vi "Configure Std Waveform.vi"(8 "error in (no error)":errorcluster, 11 "FGen PXI Base CFG in":refnum<class "FGen PXI Base CFG.lvclass">) -> (0 "error out":errorcluster, 3 "FGen PXI Base CFG out":refnum<class "FGen PXI Base CFG.lvclass">)   [LabVIEW 2023, in "FGen PXI Base CFG.lvlib" / "FGen PXI Base CFG.lvclass"]
uses:
  FGen PXI Base CFG.lvclass
  <instrlib>/niFgen/niFgen.llb/niFgen Waveform Type.ctl
  <instrlib>/niFgen/niFgen.llb/niFgen Trigger Mode.ctl
  <instrlib>/niFgen/niFgen.llb/niFgen Output Impedance.ctl
  FGen PXI Base CFG.lvclass/FGen PXI Base CFG.ctl
  Configuration/Configuration JSON/Configuration JSON Base/CFG JSON.lvclass/CFG JSON.ctl
  <instrlib>/niFgen/niFgen.llb/niFgen Output Mode.ctl
  ad788453-c75c-4861-a618-ce10b1873926.vi
  <vilib>/JDP Science/JSONtext/Find Item.vi
  <vilib>/JDP Science/JSONtext/Next JSON Value.vi
  <vilib>/JDP Science/JSONtext/String Subset.vi
  <vilib>/JDP Science/JSONtext/Parsing/Advance past next JSON Value (inlined COPY).vi
  <vilib>/JDP Science/JSONtext/Parsing/Advance past whitespace.vi
  <vilib>/JDP Science/JSONtext/Parsing/Advance past String.vi
  <vilib>/JDP Science/JSONtext/Parsing/Advance past Number.vi
  <vilib>/JDP Science/JSONtext/Parsing/Advance past Line Ending.vi
  <vilib>/JDP Science/JSONtext/Parsing/Parse Full Path or Item Name.vi
  <vilib>/JDP Science/JSONtext/Parsing/Advance past Array.vi
  <vilib>/JDP Science/JSONtext/Parsing/Advance past Object.vi
  <vilib>/JDP Science/JSONtext/support/Error Cluster From Code.vi
  <vilib>/JDP Science/JSONtext/Offset/Find Item Locations by Path.vi
  <vilib>/JDP Science/JSONtext/JSON text to Variant.vi
  <vilib>/Utility/error.llb/Error Cluster From Error Code.vi
  <vilib>/JDP Science/JSONtext/LVClass Serializer/JSONtext LVClass Serializer.lvclass
  <vilib>/ErrorRing/Error Ring.xnode
  Configuration/Configuration JSON/Configuration JSON Base/CFG JSON.lvclass
  D:/git/HAL/HAL GOOP4/FGen/FGen Base CFG/FGen Base CFG.lvclass
  D:/git/HAL/HAL GOOP4/Configuration/Configuration JSON/Configuration JSON Base/CFG JSON.lvclass
  D:/git/HAL/HAL GOOP4/Interfaces/IConfigure/IConfigure.lvclass
  D:/git/HAL/HAL GOOP4/FGen/FGen PXI/FGen PXI Base CFG/FGen PXI Base CFG.lvclass
panel:
  out "Impedance":T1 caption="Impedance (default: 0=50 ohms)" items=["50 ohms", "75 ohms"]
  out "Trigger Mode":T2 caption="Trigger Mode (default: 1=continuous)" items=["Single", "Continuous", "Stepped", "Burst"]
  out "Waveform":T3 items=["Sine", "Square", "Triangle", "Ramp Up", "Ramp Down", "DC", "Noise", "User"]
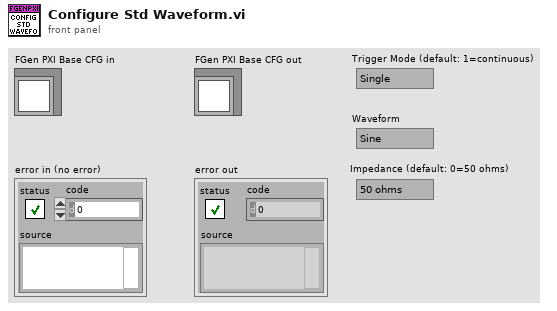
[diagram p1: front panel]
types:
  T1 = typedef "niFgen Output Impedance.ctl" = i32
  T2 = typedef "niFgen Trigger Mode.ctl" = i32
  T3 = typedef "niFgen Waveform Type.ctl" = i32
  T4 = cluster{"Name":string, "Enabled":bool, "Waveform":string, "Frequency":dbl, "Amplitude":dbl, "Start Phase":dbl, "DC Offset":dbl, "Trigger Mode":string, "Impedance":string}[]
  T5 = typedef "niFgen Output Mode.ctl" = u32
  T6 = typedef "LVStringsAndValuesArrayTypeDef_I32.ctl" = cluster{"String":string, "Value":i32}[]
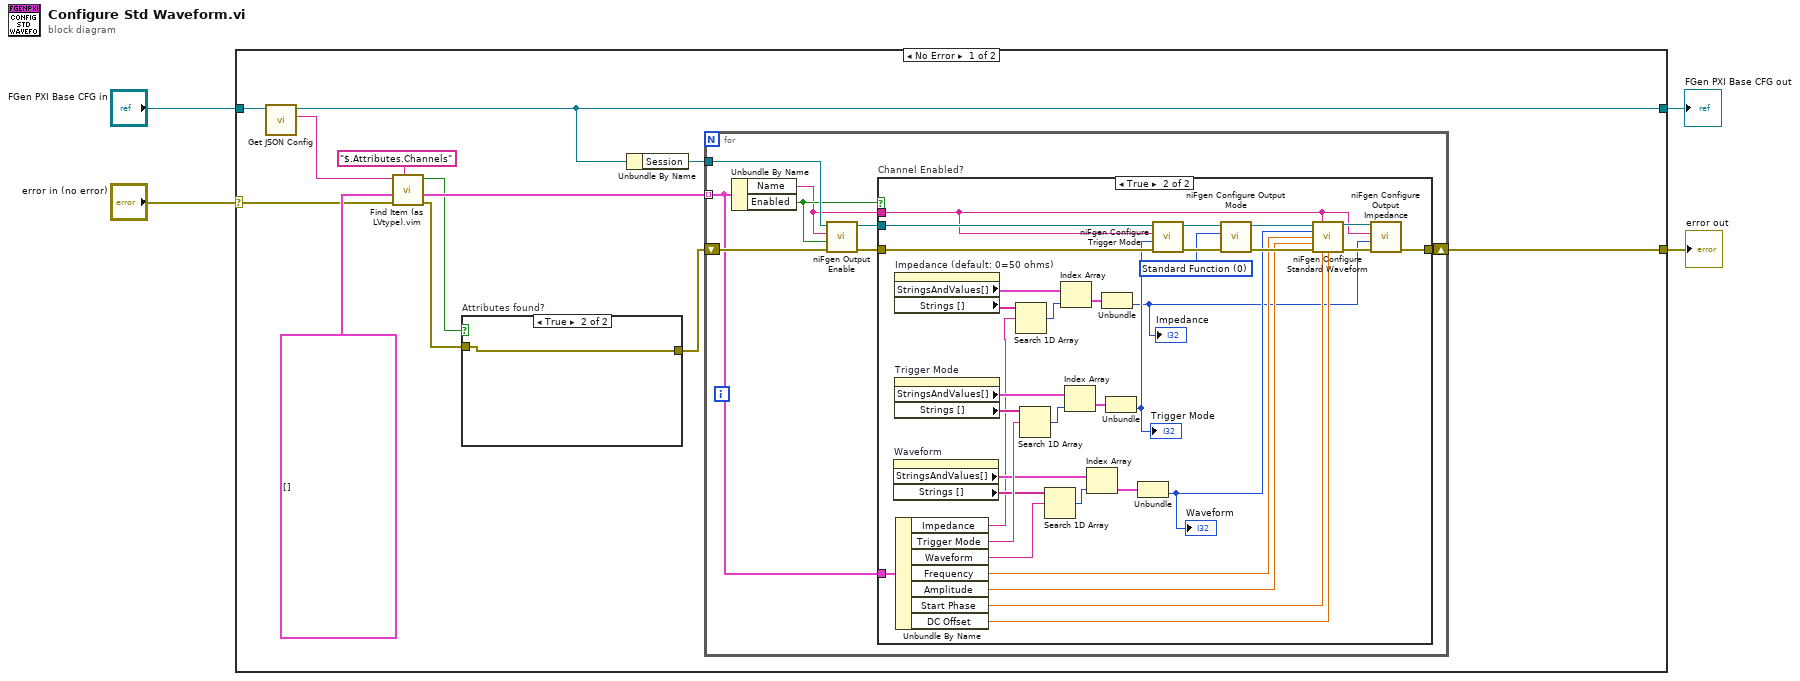
[diagram p0: block diagram]
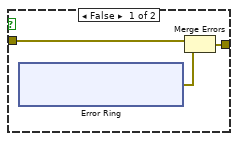
[diagram p2: hidden frame]
diagram:
  n1 = case shown="No Error" "error in (no error)" {
    selector: "error in (no error)" -> [w5 w69]
    tunnel: [w8 w70] -> w2
    tunnel: "FGen PXI Base CFG in" -> [w14 w70]
    tunnel: [w6 w69] -> w1
    frame No Error {
      n2 = call "Get JSON Config.vi"("CFG Base in"=w14) -> ("<JSON>Config>"=w13:string, "CFG Base out"=w8:refnum<class "FGen PXI Base CFG.lvclass">)  [unwired: 9 in]
      n3 = call "Find Item (as LVtype).vim"("$Path or Item Name"="$.Attributes.Channels", "error in (no error)"=w5, "Data Type and Default Value"=T4 [], "JSON"=w13) -> ("error out"=w10:errorcluster, "Data"=w12:T4, "Found"=w11:bool)  [unwired: 4 in, 1 out]
      n4 = case "Attributes found?" shown="True" w11 {
        tunnel: w10 -> [w18 w25]
        tunnel: [w17 w25] -> w9
        frame False {
          n5 = xnode "Error Ring"() -> ("error out"=w19:errorcluster)
          n6 = Merge Errors(w18, w19) -> (w17:errorcluster)
        }
        frame True {
        }
      }
      n7 = Unbundle By Name(w8) -> ("Session"=w7:refnum<k15>)
      n8 = for {
        tunnel: w12 -> [w27] mode=indexing
        tunnel: w7 -> [w32]
        shift-right: [w26] -> w6
        shift-left: w9 -> [w33]
        n9 = Unbundle By Name(w27) -> ("Name"=w28:string, "Enabled"=w31:bool)
        n10 = call <instrlib>:"niFgen Output Enable.vi"("error in (no error)"=w33, "Output Enable (default: True)"=w31, "Channel Name"=w28, "Instrument Handle"=w32) -> ("error out"=w30:errorcluster, "Instrument Handle Out"=w29:refnum<k15>)  [unwired: 6 in]
        n11 = case "Channel Enabled?" shown="True" w31 {
          tunnel: w30 -> [w34 w64]
          tunnel: w29 -> [_ w63]
          tunnel: w28 -> [_ w41]
          tunnel: w27 -> [_ w62]
          tunnel: [w34 w43] -> w26
          frame False {
          }
          frame True {
            w61 = T5 0 items=["Standard Function", "Frequency List", "Arbitrary Waveform", "Arbitrary Sequence", "Script"] ("Output Mode (default: 0=Standard Function)")
            n12 = property on="Waveform" class="Ring (strict)"() -> ("StringsAndValues[]"=w48:T6, "Strings []"=w51:string[])  [unwired: 2 in, 2 out]
            n13 = property on="Impedance (default: 0=50 ohms)" class="Ring (strict)"() -> ("StringsAndValues[]"=w38:T6, "Strings []"=w37:string[])  [unwired: 2 in, 2 out]
            n14 = property on="Trigger Mode" class="Ring (strict)"() -> ("StringsAndValues[]"=w53:T6, "Strings []"=w55:string[])  [unwired: 2 in, 2 out]
            n15 = Unbundle By Name(w62) -> ("Impedance"=w36:string, "Trigger Mode"=w54:string, "Waveform"=w50:string, "Frequency"=w60:dbl, "Amplitude"=w59:dbl, "Start Phase"=w58:dbl, "DC Offset"=w57:dbl)
            n16 = Search 1D Array(1D array=w37, element=w36) -> (index of element=w39:i32)  [unwired: 1 in]
            n17 = Search 1D Array(1D array=w55, element=w54) -> (index of element=w52:i32)  [unwired: 1 in]
            n18 = Search 1D Array(1D array=w51, element=w50) -> (index of element=w49:i32)  [unwired: 1 in]
            n19 = Index Array(array=w38, index=w39) -> (element=w40:cluster{"String":string, "Value":i32})
            n20 = Index Array(array=w53, index=w52) -> (element=w47:cluster{"String":string, "Value":i32})
            n21 = Index Array(array=w48, index=w49) -> (element=w46:cluster{"String":string, "Value":i32})
            n22 = Unbundle(w40) -> ("Value"=w35:i32)  [unwired: 1 out]
            "Impedance" <- w35
            n23 = Unbundle(w47) -> ("Value"=w45:i32)  [unwired: 1 out]
            "Trigger Mode" <- w45
            n24 = Unbundle(w46) -> ("Value"=w44:i32)  [unwired: 1 out]
            "Waveform" <- w44
            n25 = call <instrlib>:"niFgen Configure Trigger Mode.vi"("error in (no error)"=w64, "Trigger Mode (default: 1=continuous)"=w45, "Channel Name"=w41, "Instrument Handle"=w63) -> ("error out"=w67:errorcluster, "Instrument Handle Out"=w68:refnum<k15>)  [unwired: 6 in]
            n26 = call <instrlib>:"niFgen Configure Output Mode.vi"("error in (no error)"=w67, "Output Mode (default: 0=Standard Function)"=w61, "Instrument Handle"=w68) -> ("error out"=w65:errorcluster, "Instrument Handle Out"=w66:refnum<k15>)  [unwired: 6 in]
            n27 = call <instrlib>:"niFgen Configure Standard Waveform.vi"("Instrument Handle"=w66, "Channel Name"=w41, "Waveform"=w44, "Frequency"=w60, "Amplitude"=w59, "error in (no error)"=w65, "Start Phase"=w58, "DC Offset"=w57) -> ("Instrument Handle Out"=w42:refnum<k15>, "error out"=w56:errorcluster)  [unwired: 6 in]
            n28 = call <instrlib>:"niFgen Configure Output Impedance.vi"("error in (no error)"=w56, "Impedance (default: 0=50 ohms)"=w35, "Channel Name"=w41, "Instrument Handle"=w42) -> ("error out"=w43:errorcluster)  [unwired: 6 in, 1 out]
          }
        }
      }
    }
    frame Error {
    }
  }
  "error out" <- w1
  "FGen PXI Base CFG out" <- w2
